vi "sv_Enumeration (Specific Datatype).vi"() -> (2 "specific datatype strings":T1=["unknown", "general", "stress", "strain", "temperature", "heat flux", "displacement", "reaction force", "velocity", "acceleration", "excitation force", "pressure", "mass", "time", "frequency", "rpm", "order", "sound pressure", "sound intensity", "sound power"], 3 "specific datatype U16 values":u16[](array[numeric])=[0, 1, 2, 3, 5, 6, 8, 9, 11, 12, 13, 15, 16, 17, 18, 19, 20, 21, 22, 23])   [LabVIEW 2017, in "SoundVib_UFF58.lvlib"]
uses:
  <vilib>/addons/Sound and Vibration/svt_UFF58/SoundVib_UFF58.lvlib
  <vilib>/addons/Sound and Vibration/svt_UFF58/subVIs/sv_UFF58 Specific Datatype Array.ctl
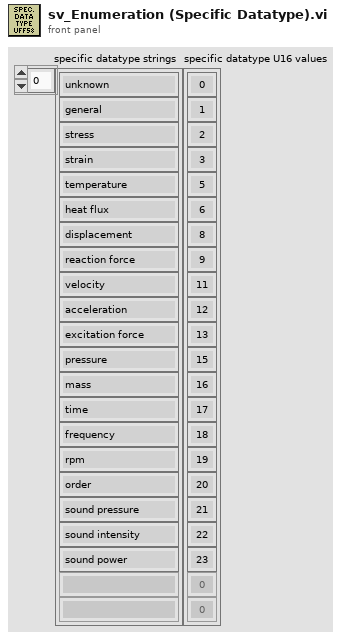
[diagram p1: front panel]
types:
  T1 = typedef "SoundVib_UFF58.lvlib/sv_UFF58 Specific Datatype Array.ctl" = string[]
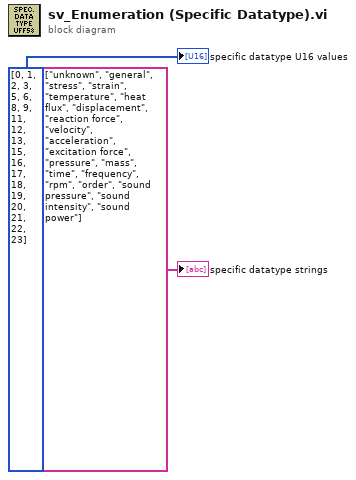
[diagram p0: block diagram]
diagram:
  "specific datatype U16 values" <- u16[] [0, 1, 2, 3, 5, 6, 8, 9, 11, 12, 13, 15, 16, 17, 18, 19, 20, 21, 22, 23] ("numeric values")
  "specific datatype strings" <- T1 ["unknown", "general", "stress", "strain", "temperature", "heat flux", "displacement", "reaction force", "velocity", "acceleration", "excitation force", "pressure", "mass", "time", "frequency", "rpm", "order", "sound pressure", "sound intensity", "sound power"] ("strings")
